vi "Post_Process_Raw_data.vi"(0 "Select Plug Ins":bool, 5 "Save results to":T1(ring)=enum."Original Results Filenames with _PP", 11 "Selected files":path[](array[path]), 12 "Current Results filenames":path[](array[path]), 13 "Results Plotter Rows":string[][](array[string])) -> ()   [LabVIEW 2011]
uses:
  Anemometry Sub Vis/Controls/File_Selector_Type.ctl
  Anemometry Sub Vis/Controls/Setup.ctl
  Anemometry Sub Vis/Controls/Save_Data.ctl
  Anemometry Sub Vis/Controls/Post_Process.ctl
  Anemometry Sub Vis/Globals/Meas_global.vi
  Anemometry Sub Vis/Globals/Plug_in_data_global.vi
panel:
  out "Single Filename":string
  out "Files not found":i32
  out "Files not Found":path[](array[path])
  out "Checking":i32
  in  "No dialogs":bool
  in  "Previous Choice":path
  in  "Search String":string
  in  "Boolean":bool
  in  "Pause Mode":enum16{"Continuous Running", "After Each File"}(ring)
  in  "At Dialog Prompt Post Process":T2=enum."All files listed in selected file"
  out "Files Processed":i32(slide) scale=0.0..1.0
  in  "stop":bool
  out "Files To Process":path[](array[path])
  in  "Post processed Results folder":path
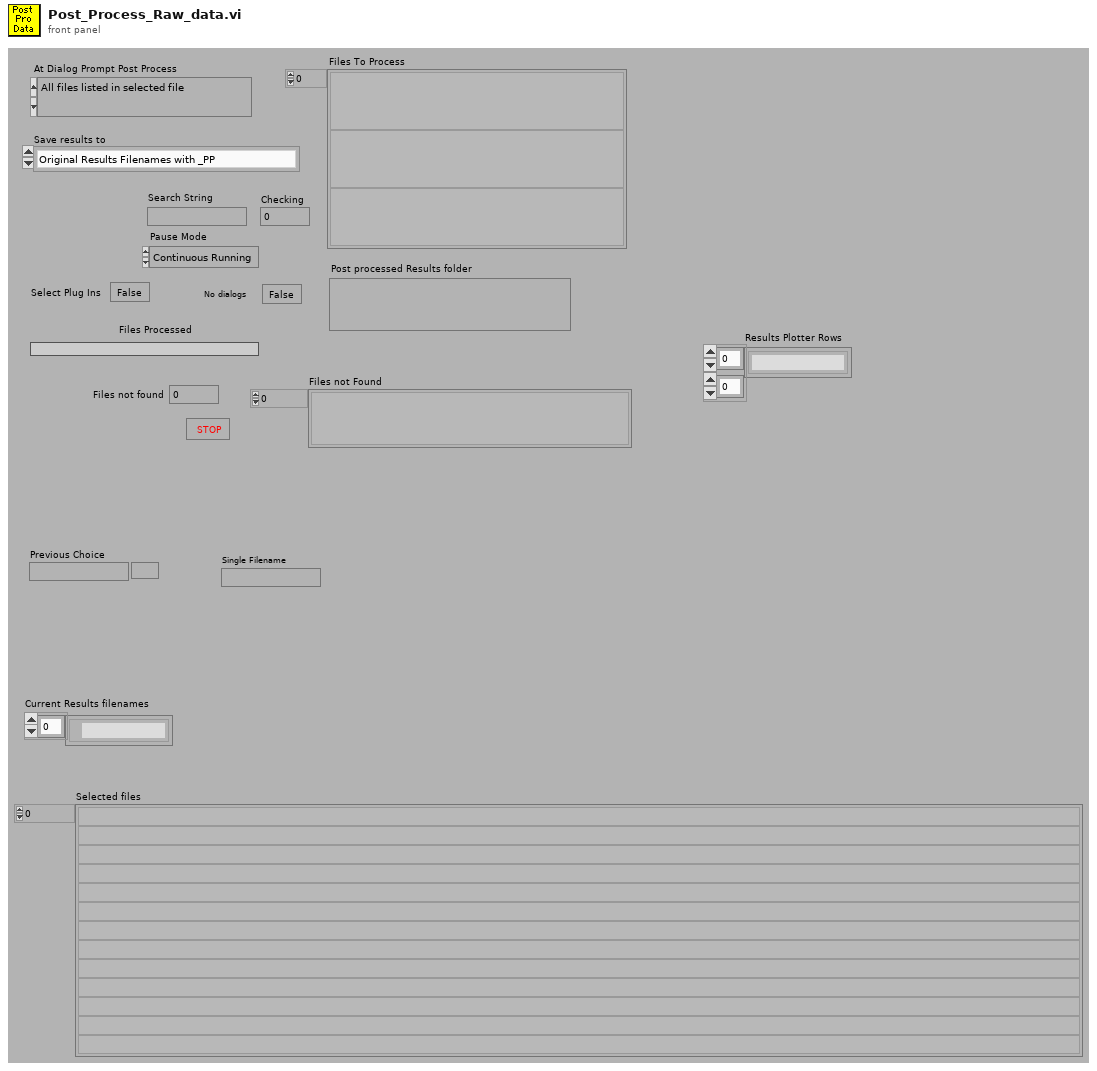
[diagram p1: front panel]
types:
  T1 = enum16{"A single file", "Original Results Filenames with _PP", "Current Results Filenames"}
  T2 = typedef "File_Selector_Type.ctl" = enum16{"The Selected File", "The Selected Folder", "Files containing the search string in the selected folder", "All files listed in selected file"}
  T3 = typedef "Setup.ctl" = enum16{"Run Program", "Show Setup", "Save Current Setup", "Setup Front Panel"}
  T4 = typedef "Save_Data.ctl" = enum16{"Save No Data", "Save Data"}
  T5 = typedef "Post_Process.ctl" = enum16{"Take New Data", "Post Process Raw Data File"}
  T6 = typedef "Multi_Run_Status.ctl" = enum16{"Continue", "Jump to Next Point", "Jump to Next Row", "Jump To Fall Back", "Terminate Run"}
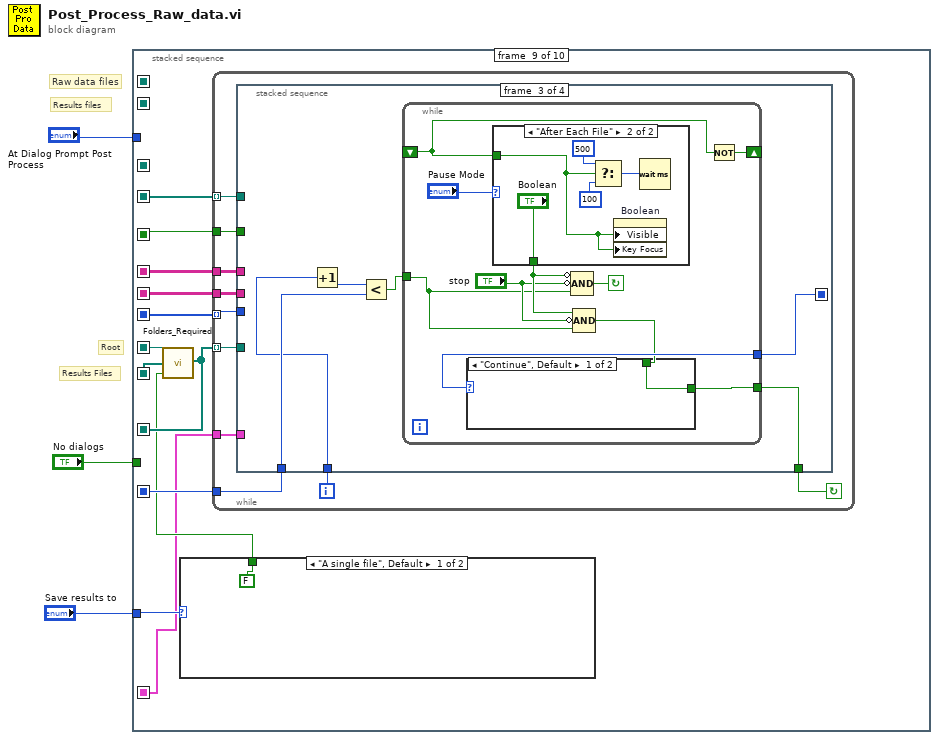
[diagram p0: block diagram]
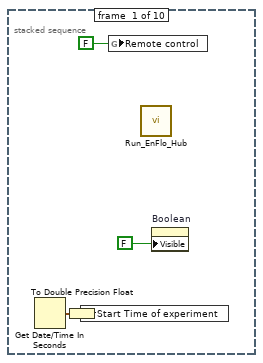
[diagram p2: hidden frame]
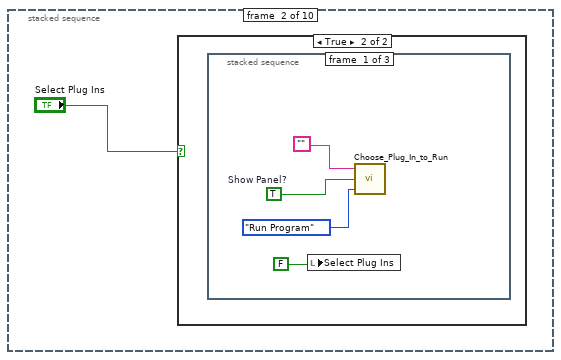
[diagram p3: hidden frame]
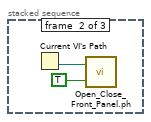
[diagram p5: hidden frame]
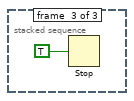
[diagram p6: hidden frame]
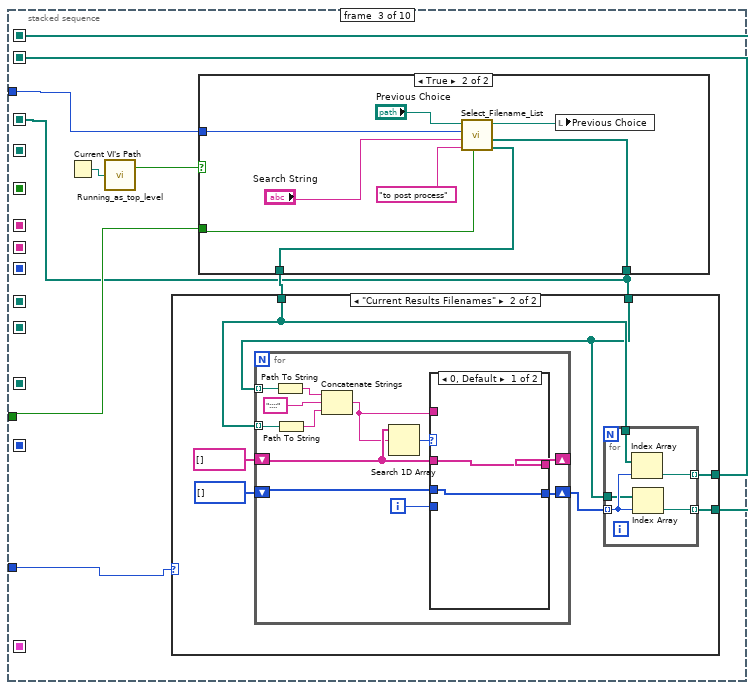
[diagram p7: hidden frame]
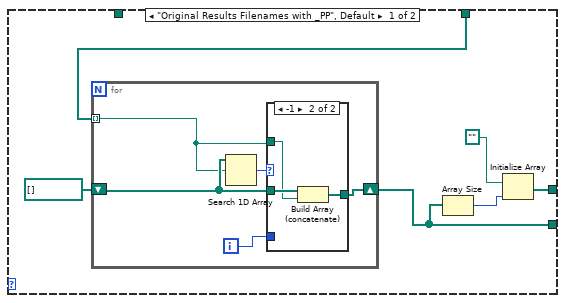
[diagram p8: hidden frame]
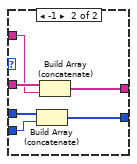
[diagram p10: hidden frame]
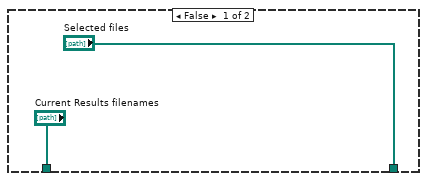
[diagram p11: hidden frame]
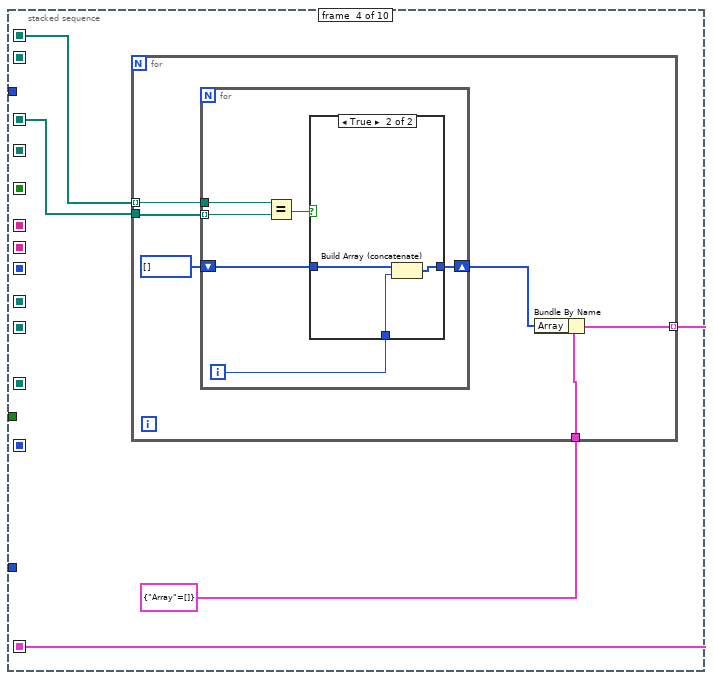
[diagram p12: hidden frame]
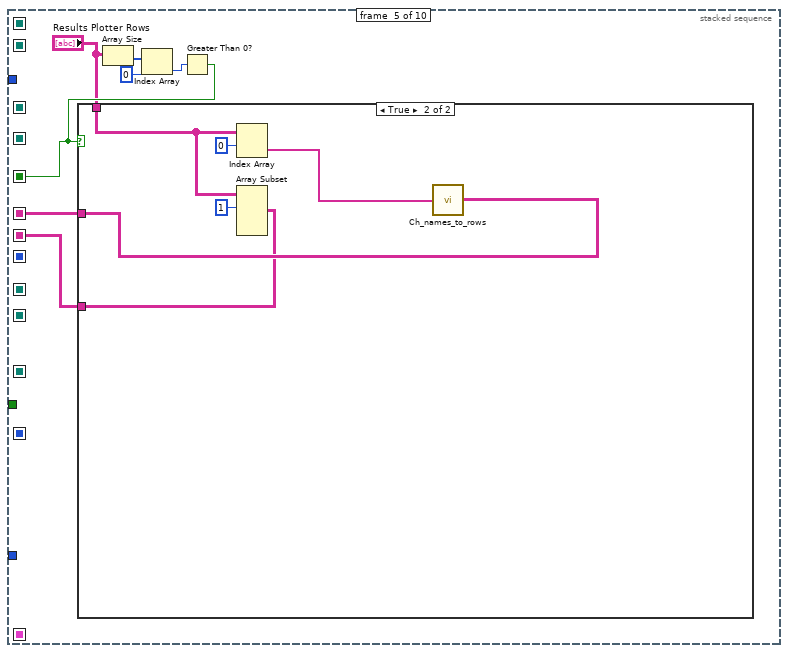
[diagram p14: hidden frame]
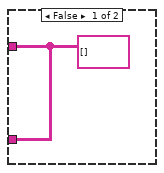
[diagram p15: hidden frame]
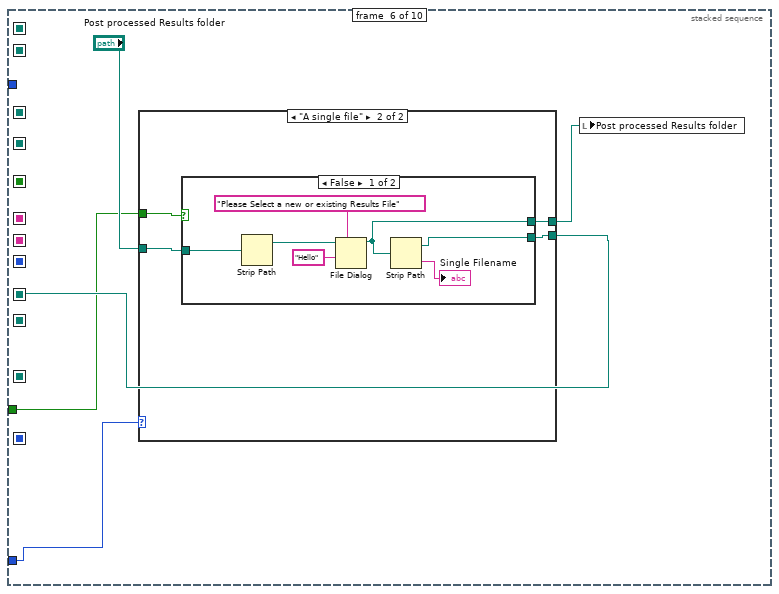
[diagram p16: hidden frame]
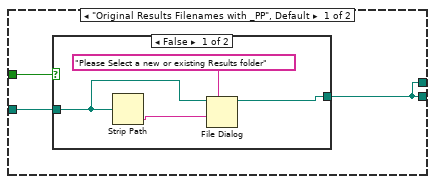
[diagram p17: hidden frame]
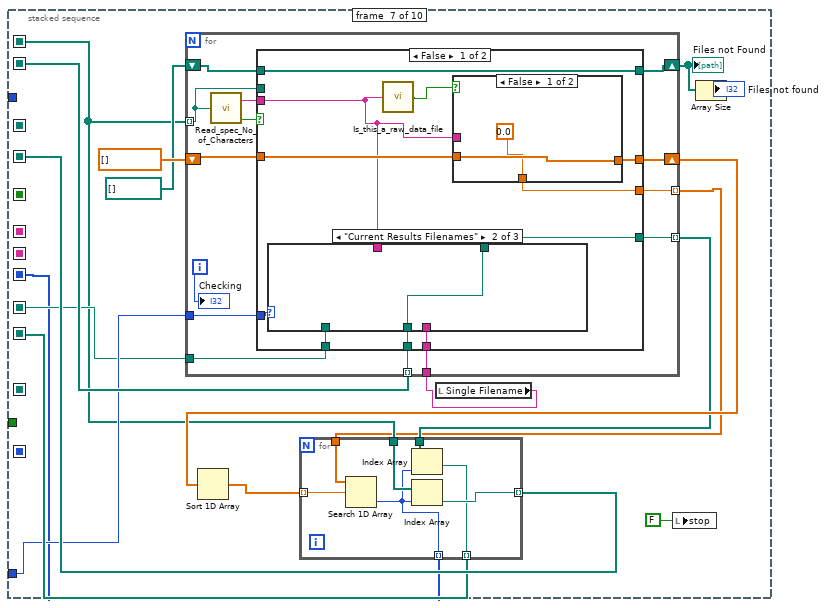
[diagram p20: hidden frame]
diagram:
  # "Results files"
  # "Raw data files"
  # "Root"
  # "Results Files"
  n1 = stacked-sequence {
    seq-local: [_ _ _ _ _ _ w154 _ _ _] -> [_ _ _ _ _ _ _ w212 w229 _]
    seq-local: [_ _ _ _ _ _ _ w217 _ _] -> [_ _ _ _ _ _ _ _ w228 _]
    seq-local: [_ _ w18 _ _ _ _ _ _ _] -> [_ _ _ w84 _ _ w143 _ _ _]
    seq-local: [_ _ _ _ _ w120 _ _ _ _] -> [_ _ _ _ _ _ w146 _ w227 _]
    seq-local: [_ _ _ _ _ _ w152 _ _ _] -> [_ _ _ _ _ _ _ _ w226 _]
    seq-local: [_ _ _ _ _ _ _ _ w225 _] -> [_ _ _ _ _ _ _ _ _ w294]
    seq-local: [_ _ w19 _ _ _ _ _ _ _] -> [_ _ _ _ _ _ w148 _ _ _]
    seq-local: [_ _ _ _ w108 _ _ _ _ _] -> [_ _ _ _ _ _ _ _ w222 _]
    seq-local: [_ _ _ _ w107 _ _ _ _ _] -> [_ _ _ _ _ _ _ _ w219 _]
    seq-local: [_ _ _ _ w103 _ _ _ _ _] -> [_ _ _ _ _ _ _ _ w221 _]
    seq-local: [_ _ _ _ _ _ w144 _ _ _] -> [_ _ _ _ _ _ _ _ w220 _]
    seq-local: [_ _ _ w82 _ _ _ _ _ _] -> [_ _ _ _ _ _ _ _ w218 _]
    seq-local: [_ _ w16 _ _ _ _ _ _ _] -> [_ _ _ w85 _ _ _ _ _ _]
    tunnel: "At Dialog Prompt Post Process" -> [_ _ w24 _ _ _ _ _ _ _]
    tunnel: "No dialogs" -> [_ _ w23 _ _ w118 _ _ _ _]
    tunnel: "Save results to" -> [_ _ w17 _ _ w117 w147 _ w224 _]
    frame #0 {
      n2 = Get Date/Time In Seconds() -> (seconds since 1Jan1904=w4:timestamp)
      n3 = To Double Precision Float(number=w4) -> (double precision float=w5:dbl)
      n4 = global write "Meas_global.vi" "Start Time of experiment"(w5) -> ()
      n5 = global write "Meas_global.vi" "Remote control"(FALSE ("Remote control")) -> ()
      n6 = call "Run_EnFlo_Hub.vi"() -> ()  [unwired: 8 out]
      n7 = property on="Boolean" class="Bool"("Visible"=FALSE ("Write Attribute")) -> ()  [unwired: 2 in, 2 out]
    }
    frame #1 {
      n8 = case shown="True" "Select Plug Ins" {
        frame False {
        }
        frame True {
          n9 = stacked-sequence {
            frame #0 {
              w12 = TRUE  # Show Panel?
              n10 = local write "Select Plug Ins"(FALSE ("Select Local ADAM Channels")) -> ()
              n11 = call "Choose_Plug_In_to_Run.vi"("setup"=Setup."Run Program", "Show Panel?"=w12, "Setup String In"="") -> ()  [unwired: 2 out]
            }
            frame #1 {
              n12 = Current VI's Path() -> (path=w14:path)
              n13 = call "Open_Close_Front_Panel.ph.vi"("Front Panel Window:Open"=TRUE, "VI path"=w14) -> ()  [unwired: 2 out]
            }
            frame #2 {
              n14 = Stop(stop? (T)=TRUE) -> ()
            }
          }
        }
      }
    }
    frame #2 {
      n15 = Current VI's Path() -> (path=w22:path)
      n16 = call "Running_as_top_level.vi"("Vi path name"=w22) -> ("Top Level"=w21:bool)  [unwired: 1 out]
      n17 = case shown="True" w21 {
        tunnel: w24 -> [_ w81]
        tunnel: w23 -> [_ w76]
        tunnel: ["Selected files" w75] -> w16
        tunnel: ["Current Results filenames" w74] -> w20
        frame False {
        }
        frame True {
          n18 = call "Select_Filename_List.vi"("No dialogs"=w76, "File Type"="to post process", "Search String"="Search String", "At Dialog Prompt Post Process"=w81, "Previous Choice"="Previous Choice") -> ("Current Results filenames"=w74:path[], "Selected files"=w75:path[], "Choosen path"=w77:path)  [unwired: 1 out]
          n19 = local write "Previous Choice"(w77) -> ()
        }
      }
      n20 = case shown="\"Current Results Filenames\"" w17 {
        tunnel: w16 -> [w30 w43]
        tunnel: w20 -> [_ w44]
        tunnel: [w26 w42] -> w19
        tunnel: [w28 w41] -> w18
        frame "Original Results Filenames with _PP", Default {
          n21 = for {
            shift-right: [w34] -> w28
            shift-left: path[] [] -> [w35]
            tunnel: w30 -> [w31] mode=indexing
            i -> [w32]
            n22 = Search 1D Array(1D array=w35, element=w31) -> (index of element=w33:i32)  [unwired: 1 out]
            n23 = case shown="-1" w33 {
              tunnel: w35 -> [w36 w39]
              tunnel: [w36 w38] -> w34
              tunnel: w31 -> [_ w37]
              tunnel: w32 -> [_ _]
              frame 0, Default {
              }
              frame -1 {
                n24 = Build Array (concatenate)(w39, w37) -> (w38:path[])
              }
            }
          }
          n25 = Array Size(array=w28) -> (size(s)=w27:i32)
          n26 = Initialize Array(path "", w27) -> (w26:path[])
        }
        frame "Current Results Filenames" {
          n27 = for {
            shift-right: [w62] -> _
            shift-left: string[] [] -> [w63]
            tunnel: w43 -> [w61] mode=indexing
            tunnel: w44 -> [w55] mode=indexing
            shift-right: [w57] -> w40
            shift-left: i32[] [] -> [w56]
            i -> [w58]
            n28 = Path To String(path=w61) -> (string=w60:string)
            n29 = Path To String(path=w55) -> (string=w54:string)
            n30 = Concatenate Strings(w60, "::::" ("string"), w54) -> (w53:string)
            n31 = Search 1D Array(1D array=w63, element=w53) -> (index of element=w52:i32)  [unwired: 1 out]
            n32 = case shown="0, Default" w52 {
              tunnel: w63 -> [w65 w71]
              tunnel: [w65 w70] -> w62
              tunnel: w53 -> [_ w67]
              tunnel: w58 -> [_ w66]
              tunnel: [w64 w69] -> w57
              tunnel: w56 -> [w64 w68]
              frame 0, Default {
              }
              frame -1 {
                n33 = Build Array (concatenate)(w68, w66) -> (w69:i32[])
                n34 = Build Array (concatenate)(w71, w67) -> (w70:string[])
              }
            }
          }
          n35 = for {
            tunnel: w40 -> [w51] mode=indexing
            tunnel: w44 -> [w50]
            tunnel: w43 -> [w49]
            tunnel: [w48] -> w42 mode=indexing
            tunnel: [w47] -> w41 mode=indexing
            n36 = Index Array(array=w50, index=w51) -> (element=w48:path)
            n37 = Index Array(array=w49, index=w51) -> (element=w47:path)
          }
        }
      }
    }
    frame #3 {
      n38 = for {
        tunnel: w85 -> [w90]
        tunnel: w84 -> [w91] mode=indexing
        tunnel: cluster{"Array":i64[]} {"Array"=[]} ("Cluster") -> [w88]
        tunnel: [w86] -> w82 mode=indexing
        n39 = for {
          tunnel: w91 -> [w97]
          tunnel: w90 -> [w96] mode=indexing
          shift-right: [w93] -> w87
          shift-left: i32[] [] -> [w94]
          i -> [w92]
          n40 = Equal?(x=w97, y=w96) -> (x = y?=w95:bool)
          n41 = case shown="True" w95 {
            tunnel: w94 -> [w98 w101]
            tunnel: [w98 w100] -> w93
            tunnel: w92 -> [_ w99]
            frame False {
            }
            frame True {
              n42 = Build Array (concatenate)(w101, w99) -> (w100:i32[])
            }
          }
        }
        n43 = Bundle By Name(cluster=w88, "Array"=w87) -> (w86:cluster{"Array":i64[]})
      }
    }
    frame #4 {
      n44 = Array Size(array="Results Plotter Rows") -> (size(s)=w106:i32[])
      n45 = Index Array(array=w106, index=0) -> (element=w104:i32)
      n46 = Greater Than 0?(x=w104) -> (x > 0?=w103:bool)
      n47 = case shown="True" w103 {
        tunnel: [w109 w115] -> w108
        tunnel: [w109 w110] -> w107
        tunnel: "Results Plotter Rows" -> [_ w113]
        frame False {
          w109 = string[][] [] ("3 Row names")
        }
        frame True {
          n48 = Index Array(array=w113, index (row)=0 ("index")) -> (element=w111:string[])  [unwired: 1 in]
          n49 = Array Subset(array=w113, index (row)=1 ("index")) -> (w110:string[][])  [unwired: 3 in]
          n50 = call "Ch_names_to_rows.vi"("Channel Names"=w111) -> ("3 Row names"=w115:string[][])
        }
      }
    }
    frame #5 {
      n51 = case shown="\"A single file\"" w117 {
        tunnel: [w121 w132] -> w120
        tunnel: "Post processed Results folder" -> [w123 w131]
        tunnel: w118 -> [w122 w130]
        tunnel: [w121 w129] -> w116
        frame "Original Results Filenames with _PP", Default {
          n52 = case shown="False" w122 {
            tunnel: [w127 w128] -> w121
            tunnel: w123 -> [w124 w128]
            frame False {
              n53 = Strip Path(path=w124) -> (name=w125:string)  [unwired: 1 out]
              n54 = File Dialog(7:"Please Select a new or existing Results folder" ("prompt"), 9:w125, 11:w124) -> (3:w127:path)  [unwired: 1 in, 6 out]
            }
            frame True {
            }
          }
        }
        frame "A single file" {
          n55 = case shown="False" w130 {
            tunnel: [w138 w140] -> w132
            tunnel: w131 -> [w136 w140]
            tunnel: [w135 w140] -> w129
            frame False {
              n56 = Strip Path(path=w136) -> (stripped path=w134:path)  [unwired: 1 out]
              n57 = File Dialog(7:"Please Select a new or existing Results File" ("prompt"), 9:"Hello" ("default name"), 11:w134) -> (3:w135:path)  [unwired: 1 in, 6 out]
              n58 = Strip Path(path=w135) -> (stripped path=w138:path, name=→"Single Filename":string)
            }
            frame True {
            }
          }
        }
      }
      n59 = local write "Post processed Results folder"(w116) -> ()
    }
    frame #6 {
      n60 = local read "Single Filename"() -> (w145:string)
      n61 = for {
        tunnel: w143 -> [w173] mode=indexing
        shift-right: [w177] -> w157
        shift-left: dbl[] [] -> [w178]
        shift-right: [w174] -> w150
        shift-left: path[] [] -> [w175]
        tunnel: w148 -> [w170] mode=indexing
        tunnel: w147 -> [w169]
        tunnel: w146 -> [w168]
        tunnel: w145 -> [w167]
        tunnel: [w166] -> w142 mode=indexing
        tunnel: [w165] -> w141 mode=indexing
        i -> [w176]
        n62 = call "Read_spec_No_of_Characters.vi"("Filename"=w173) -> ("character string"=w172:string, "Error?"=w171:bool)
        n63 = case shown="False" w171 {
          tunnel: w178 -> [w189 w211]
          tunnel: [w188 w211] -> w177
          tunnel: w173 -> [_ w209]
          tunnel: w175 -> [w186 w210]
          tunnel: [w186 w208] -> w174
          tunnel: w172 -> [w185 _]
          tunnel: w170 -> [w183 w207]
          tunnel: w169 -> [w184 _]
          tunnel: w168 -> [w182 _]
          tunnel: w167 -> [w181 _]
          tunnel: [w180 w207] -> w166
          tunnel: [w179 0.0 ("Value")] -> w165
          frame False {
            n64 = case shown="\"Current Results Filenames\"" w184 {
              tunnel: [w192 w193 w196] -> w180
              tunnel: w185 -> [_ _ w194]
              tunnel: w183 -> [_ w193 _]
              tunnel: w182 -> [w191 _ _]
              tunnel: w181 -> [w190 _ _]
              frame "A single file" {
                n65 = Build Path(base path=w191, name or relative path=w190) -> (appended path=w192:path)
              }
              frame "Current Results Filenames" {
              }
              frame "Original Results Filenames with _PP" {
                w197 = FALSE  # Show Dialog?
                n66 = call "Get_Characters_from_string.vi"("Show Dialog?"=w197, "Input string"=w194, "Variable name"="Results filename") -> ("Value"=w195:string)  [unwired: 1 out]
                n67 = call "String_to_Pathname.vi"("Input String"=w195) -> ("path"=w196:path)
              }
            }
            n68 = call "Is_this_a_raw_data_file.vi"("character string"=w185) -> ("Raw Dat File?"=w187:bool)  [unwired: 2 out]
            n69 = case shown="False" w187 {
              tunnel: w189 -> [w200 w202]
              tunnel: [w200 w205] -> w188
              tunnel: w185 -> [_ w203]
              tunnel: [0.0 ("Value") w201] -> w179
              frame False {
              }
              frame True {
                n70 = call "Get_value_from_string.vi"("Input string"=w203, "Variable name"="Seconds since 1/1/04") -> ("Value"=w201:dbl)  [unwired: 1 in, 1 out]
                n71 = Build Array (concatenate)(w202, w201) -> (w205:dbl[])
              }
            }
          }
          frame True {
            n72 = Build Array (concatenate)(w210, w209) -> (w208:path[])
          }
        }
        "Checking" <- w176
      }
      "Files not Found" <- w150
      n73 = Sort 1D Array(array=w157) -> (sorted array=w156:dbl[])
      n74 = for {
        tunnel: w141 -> [w164]
        tunnel: w156 -> [w163] mode=indexing
        tunnel: w143 -> [w162]
        tunnel: [w161] -> w154 mode=indexing
        tunnel: w142 -> [w160]
        tunnel: [w159] -> w152 mode=indexing
        tunnel: [w158] -> w144 mode=indexing
        n75 = Search 1D Array(1D array=w164, element=w163) -> (index of element=w158:i32)  [unwired: 1 out]
        n76 = Index Array(array=w160, index=w158) -> (element=w159:path)
        n77 = Index Array(array=w162, index=w158) -> (element=w161:path)
      }
      n78 = local write "stop"(FALSE ("stop")) -> ()
      n79 = Array Size(array=w150) -> (size(s)=→"Files not found":i32)
    }
    frame #7 {
      w213 = 0 ("Files Processed")
      n80 = Array Size(array=w212) -> (size(s)=w217:i32)
      n81 = Array Size(array=w212) -> (size(s)=w215:i32)
      n82 = property on="Files Processed" class="Slide (strict)"("Scale.Range:Minimum"=0.0 ("Write Attribute"), "Scale.Range:Maximum"=w215) -> ()  [unwired: 2 in, 2 out]
      n83 = local write "Files Processed"(w213) -> ()
      n84 = Build Array(w213) -> (w214:i32[])
      n85 = property on="Attribute Node" class="Arr (strict)"("Index Values"=w214) -> ()  [unwired: 2 in, 2 out]
      "Files To Process" <- w212
    }
    frame #8 {
      n86 = case shown="\"A single file\", Default" w224 {
        tunnel: [FALSE TRUE] -> w223
        frame "A single file", Default {
        }
        frame "Original Results Filenames with _PP" {
        }
      }
      n87 = call "Folders_Required.vi"("Add _pp?"=w223, "Filenames"=w226, "New Root"=w227) -> ("Array"=w225:path[])
      n88 = while {
        tunnel: w225 -> [w237] mode=indexing
        tunnel: w228 -> [w240]
        tunnel: w229 -> [w241] mode=indexing
        tunnel: w222 -> [w236]
        tunnel: w220 -> [w233] mode=indexing
        tunnel: w221 -> [w235]
        tunnel: w219 -> [w234]
        tunnel: w218 -> [w232]
        i -> [w239]
        stop <- w238 continue-if-true
        n89 = stacked-sequence {
          seq-local: [_ w263 _ _] -> [_ _ w267 _]
          tunnel: w237 -> [_ w265 _ _]
          tunnel: w241 -> [_ w264 _ _]
          tunnel: w240 -> [_ _ w269 _]
          tunnel: w239 -> [_ _ w268 w291]
          tunnel: [_ _ w266 _] -> w238
          tunnel: w236 -> [w250 _ _ _]
          tunnel: w235 -> [w249 _ _ _]
          tunnel: w234 -> [w245 _ _ _]
          tunnel: w233 -> [w246 _ _ _]
          tunnel: w232 -> [w247 _ _ _]
          frame #0 {
            n90 = Index Array(array=w247, index=w246) -> (element=w244:cluster{"Array":i64[]})
            n91 = Unbundle By Name(w244) -> ("Array"=w243:i64[])
            n92 = for {
              tunnel: w245 -> [w253]
              tunnel: w243 -> [w252] mode=indexing
              tunnel: [w251] -> w242 mode=indexing
              n93 = Index Array(array=w253, index (row)=w252) -> (element=w251:string[])  [unwired: 1 in]
            }
            n94 = case shown="True" w249 {
              tunnel: w250 -> [_ w257]
              tunnel: w242 -> [_ w256]
              tunnel: ["" w255] -> w248
              frame False {
              }
              frame True {
                n95 = Build Array (concatenate)(w257, w256) -> (w259:string[][])
                n96 = Array To Spreadsheet String(array=w259, 3:"%s" ("format string")) -> (spreadsheet string=w255:string)  [unwired: 1 out]
              }
            }
            n97 = global write "Plug_in_data_global.vi" "Templated Results header"(w248) -> ()
          }
          frame #1 {
            n98 = call "Measurement.vi"("setup"=Setup."Run Program", "Post Process"=Post_Process."Post Process Raw Data File", "File"=Save_Data."Save Data", "Results file"=w265, "Raw data file"=w264) -> ("Status Out"=w263:T6)  [unwired: 2 in, 12 out]
          }
          frame #2 {
            n99 = Increment(x=w268) -> (x+1=w271:i32)
            n100 = Less?(x=w271, y=w269) -> (x < y?=w270:bool)
            n101 = while {
              shift-left: _ -> [w277]
              shift-right: [w278] -> _
              tunnel: [w280] -> w266
              tunnel: w267 -> [w281]
              tunnel: w270 -> [w273]
              stop <- w276 continue-if-true
              n102 = case shown="\"After Each File\"" "Pause Mode" {
                tunnel: [TRUE "Boolean"] -> w275
                tunnel: w277 -> [_ w286]
                frame "Continuous Running" {
                }
                frame "After Each File" {
                  n103 = Select(t=u32 500 ("milliseconds to wait"), s=w286, f=u32 100) -> (s? t:f=w283:u32)
                  n104 = property on="Boolean" class="Bool"("Visible"=w286, "Key Focus"=w286) -> ()  [unwired: 2 in, 2 out]
                  n105 = Wait (ms)(milliseconds to wait=w283) -> ()  [unwired: 1 out]
                }
              }
              n106 = Compound Arithmetic op=AND(invert w275, invert "stop", w273) -> (w276:bool)
              n107 = Compound Arithmetic op=AND(w275, invert "stop", w273) -> (w272:bool)
              n108 = case shown="\"Continue\", Default" w281 {
                tunnel: [w288 FALSE] -> w280
                tunnel: w272 -> [w288 _]
                frame "Continue", Default {
                }
                frame "Terminate Run" {
                }
              }
              n109 = Not(x=w277) -> (.not. x?=w278:bool)
            }
          }
          frame #3 {
            n110 = Increment(x=w291) -> (x+1=w290:i32)
            "Files Processed" <- w290
            n111 = Build Array(w290) -> (w292:i32[])
            n112 = property on="Attribute Node" class="Arr (strict)"("Index Values"=w292) -> ()  [unwired: 2 in, 2 out]
          }
        }
      }
    }
    frame #9 {
      n113 = Path To String(path=w294) -> (string=w296:string[])
      n114 = call "Analyse_string_array.vi"("String array"=w296) -> ("Unique strings"=w295:string[])  [unwired: 2 out]
      n115 = String To Path(string=w295) -> (path=w293:path[])
      n116 = for {
        tunnel: w293 -> [w300] mode=indexing
        w301 = FALSE  # Lock File
        n117 = call "Lock_File.vi"("Lock File"=w301, "path"=w300) -> ()  [unwired: 1 in, 3 out]
      }
      n118 = Build Array(0) -> (w298:i32[])
      n119 = property on="Boolean" class="Bool"("Visible"=FALSE ("Write Attribute")) -> ()  [unwired: 2 in, 2 out]
      n120 = property on="Attribute Node" class="Arr (strict)"("Index Values"=w298) -> ()  [unwired: 2 in, 2 out]
    }
  }
